vi "Dequeue Queue.vi"(8 "Error In":errorcluster, 11 "Queue Ref In":refnum<queue>) -> (0 "Error Out":errorcluster, 1 "Data":variant, 2 "Dequeue":string, 3 "Queue Ref Out":refnum<queue>)   [LabVIEW 2016, in "SLL QSM.lvlib"]
doc: "Dequeues an element from the Queue"
uses:
  SLL QSM.lvlib
  Typedefs/Queue Type.ctl
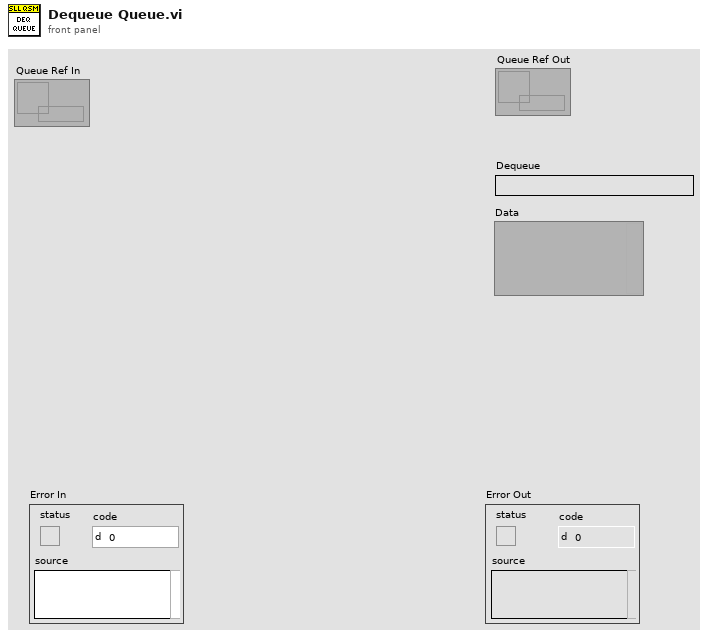
[diagram p1: front panel]
types:
  T1 = typedef "SLL QSM.lvlib/Queue Type.ctl" = cluster{"State":string, "Data":variant}
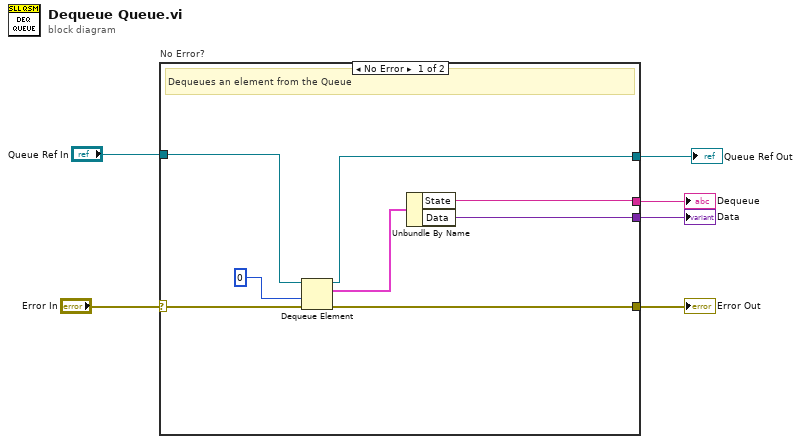
[diagram p0: block diagram]
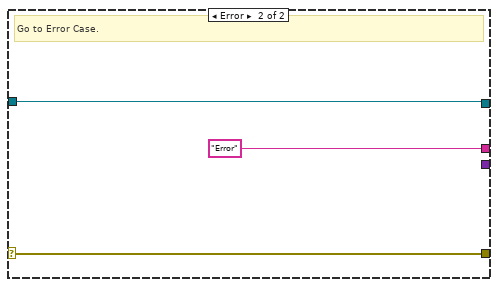
[diagram p2: hidden frame]
diagram:
  n1 = case "No Error?" shown="No Error" "Error In" {
    selector: "Error In" -> [w9 w17]
    tunnel: [w14 w17] -> w6
    tunnel: [w11 "Error" ("State In")] -> w5
    tunnel: [w10 _] -> w3
    tunnel: "Queue Ref In" -> [w8 w15]
    tunnel: [w7 w15] -> w1
    frame No Error {
      # "Dequeues an element from the Queue"
      n2 = Dequeue Element(queue=w8, timeout in ms (-1)=0, error in (no error)=w9) -> (queue out=w7:refnum<queue>, element=w12:T1, error out=w14:errorcluster)  [unwired: 1 out]
      n3 = Unbundle By Name(w12) -> ("State"=w11:string, "Data"=w10:variant)
    }
    frame Error {
      # "Go to Error Case."
    }
  }
  "Dequeue" <- w5
  "Error Out" <- w6
  "Data" <- w3
  "Queue Ref Out" <- w1
